vi "array.vi"() -> ()   [LabVIEW 2015]
uses:
  Control 1.ctl
panel:
  out "index of element":i32
  in  "search element":dbl
  out "size(s)":i32
  out "transposed array":T1[][](array[typedef])
  in  "Array 2":T1[][](array[typedef])
  out "min value":dbl
  out "max value":dbl
  out "Sorted Array":dbl[](array[numeric])
  in  "Array":dbl[](array[numeric])
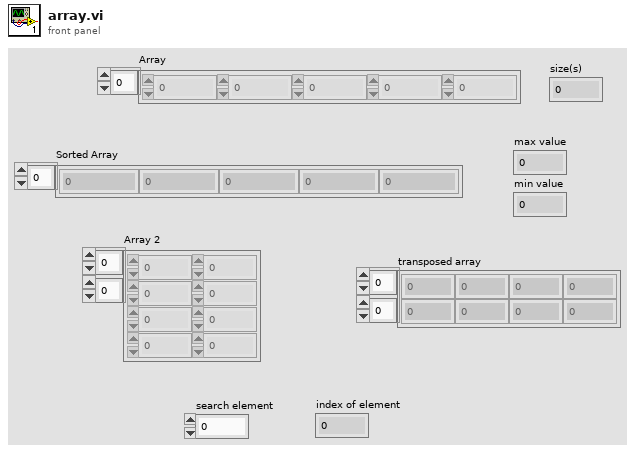
[diagram p1: front panel]
types:
  T1 = typedef "Control 1.ctl" = dbl
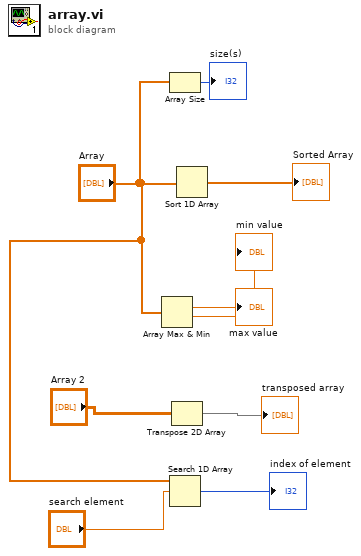
[diagram p0: block diagram]
diagram:
  n1 = Array Max & Min(array="Array") -> (max value=→"max value":dbl, min value=→"min value":dbl)  [unwired: 2 out]
  n2 = Array Size(array="Array") -> (size(s)=→"size(s)":i32)
  n3 = Search 1D Array(1D array="Array", element="search element") -> (index of element=→"index of element":i32)  [unwired: 1 in]
  n4 = Transpose 2D Array(2D array="Array 2") -> (transposed array=→"transposed array":T1[][])
  n5 = Sort 1D Array(array="Array") -> (sorted array=→"Sorted Array":dbl[])
